vi "Python_Close.vi"(8 "error in (no error) 2":errorcluster) -> (0 "error out":errorcluster)   [LabVIEW 2021]
doc: "This example demonstrates how to call a Python function and pass integers as arguments. It uses a python function to compute the sum of two integers."
uses:
  Global_Variables.vi
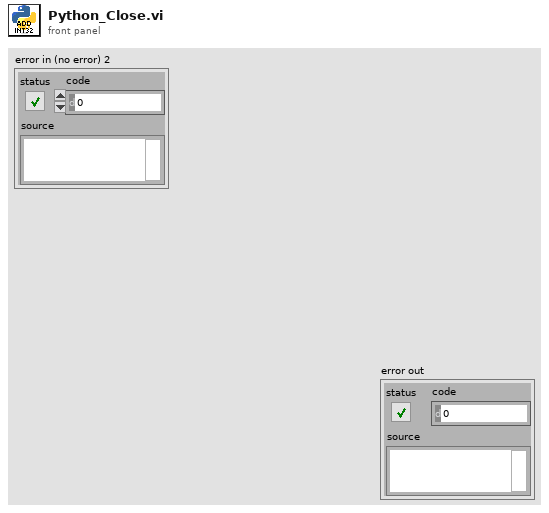
[diagram p1: front panel]
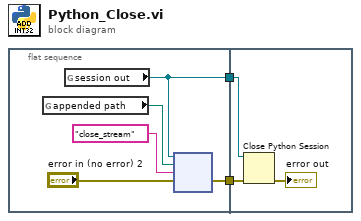
[diagram p0: block diagram]
diagram:
  n1 = flat-sequence {
    tunnel: [w5] -> w2
    tunnel: [w3] -> w1
    tunnel: w2 -> [w9]
    tunnel: w1 -> [w8]
    frame #0 {
      n2 = global read "Global_Variables.vi" "appended path"() -> (w4:path)
      n3 = global read "Global_Variables.vi" "session out"() -> (w3:refnum<k35>)
      n4 = node(w3, w4, "close_stream" ("function name"), "error in (no error) 2") -> (w5:errorcluster)  [unwired: 2 in, 3 out]
    }
    frame #1 {
      n5 = Close Python Session(session in=w8, error in=w9) -> (11:→"error out":errorcluster)
    }
  }
